vi "hmi_store_data.vi"(10 "data_store_mode":enum16{"Set", "Get"}(ring), 11 "UserData":T1) -> (3 "UserData out":T1)   [LabVIEW 2011]
uses:
  user_data.ctl
  user_buttons_dualaction.ctl
  user_buttons_360.ctl
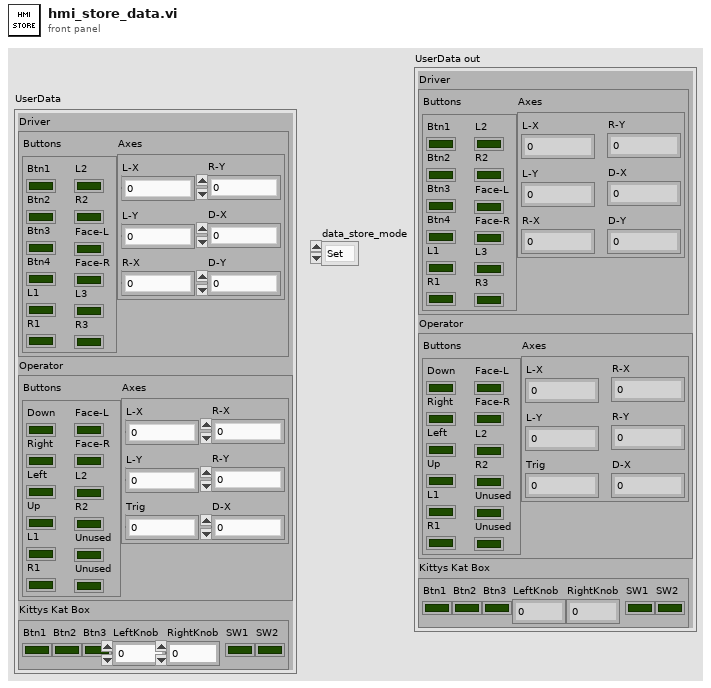
[diagram p1: front panel]
types:
  T1 = typedef "user_data.ctl" = cluster{"Driver":cluster{"Buttons":T2, "Axes":cluster{"L-X":dbl, "L-Y":dbl, "R-X":dbl, "R-Y":dbl, "D-X":dbl, "D-Y":dbl}}, "Operator":cluster{"Buttons":T3, "Axes":cluster{"L-X":dbl, "L-Y":dbl, "Trig":dbl, "R-X":dbl, "R-Y":dbl, "D-X":dbl}}, "Kittys Kat Box":cluster{"Btn1":bool, "Btn2":bool, "Btn3":bool, "LeftKnob":dbl, "RightKnob":dbl, "SW1":bool, "SW2":bool}}
  T2 = typedef "user_buttons_dualaction.ctl" = cluster{"Btn1":bool, "Btn2":bool, "Btn3":bool, "Btn4":bool, "L1":bool, "R1":bool, "L2":bool, "R2":bool, "Face-L":bool, "Face-R":bool, "L3":bool, "R3":bool}
  T3 = typedef "user_buttons_360.ctl" = cluster{"Down":bool, "Right":bool, "Left":bool, "Up":bool, "L1":bool, "R1":bool, "Face-L":bool, "Face-R":bool, "L2":bool, "R2":bool, "Unused":bool, "Unused":bool}
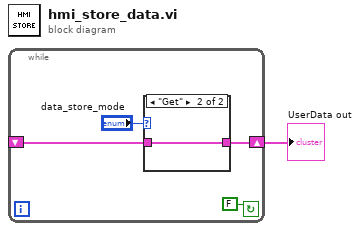
[diagram p0: block diagram]
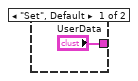
[diagram p2: hidden frame]
diagram:
  n1 = while {
    shift-right: [w3] -> w1
    shift-left: _ -> [w2]
    stop <- FALSE continue-if-true
    n2 = case shown="\"Get\"" "data_store_mode" {
      tunnel: ["UserData" w7] -> w3
      tunnel: w2 -> [_ w7]
      frame "Set", Default {
      }
      frame "Get" {
      }
    }
  }
  "UserData out" <- w1
